vi "4_Wire_Resistance.vi"(6 "Waveform_Template":waveform(dbl), 8 "error in":errorcluster, 11 "DAQ970 in":refnum<class "DAQ970.lvclass">) -> (0 "error out":errorcluster, 2 "Resistive_Measurement":waveform(dbl)[](array[waveform]), 3 "DAQ970 out":refnum<class "DAQ970.lvclass">)   [LabVIEW 2019, in "DAQ970.lvlib" / "DAQ970.lvclass"]
uses:
  Library/DAQ970.lvclass
  Library/DAQ970.lvclass/DAQ970.ctl
  <instrlib>/Keysight DAQ970/Keysight DAQ970.lvlib
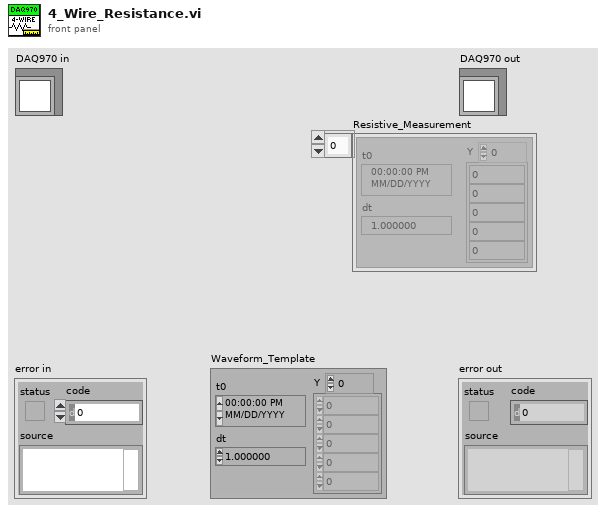
[diagram p1: front panel]
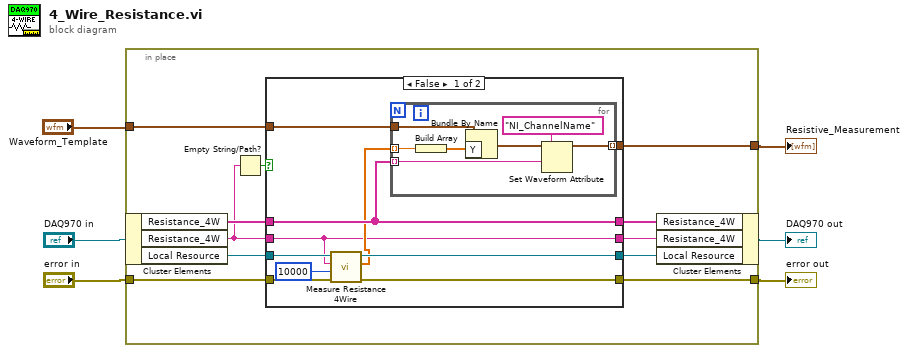
[diagram p0: block diagram]
diagram:
  n1 = in-place {
    in-place-border: "error in" -> [w11]
    in-place-border: [w12] -> w4
    in-place-border: "Waveform_Template" -> [w17]
    in-place-border: [w15] -> w6
    n2 = in-place-cluster #1("DAQ970 in") -> ("Resistance_4W"=w16:string[], "Resistance_4W"=w10:string, "Local Resource"=w14:refnum<k15>)
    n3 = Empty String/Path?(string/path=w10) -> (empty?=w9:bool)
    n4 = case shown="False" w9 {
      tunnel: w17 -> [w27 _]
      tunnel: w16 -> [w25 w38]
      tunnel: [w26 _] -> w15
      tunnel: w14 -> [w24 w36]
      tunnel: [w23 w36] -> w13
      tunnel: [w21 w35] -> w12
      tunnel: w11 -> [w20 w35]
      tunnel: w10 -> [w18 w37]
      tunnel: [w25 w38] -> w8
      tunnel: [w18 w37] -> w7
      frame False {
        n5 = call <instrlib>:"Measure Resistance 4Wire.vi"("error in (no error)"=w20, "MaxTimeMilliseconds"=10000, "ChannelList"=w18, "instrument handle"=w24) -> ("error out"=w21:errorcluster, "Val"=w22:dbl[], "instrument handle out"=w23:refnum<k15>)  [unwired: 4 in, 1 out]
        n6 = for {
          tunnel: w22 -> [w33] mode=indexing
          tunnel: w27 -> [w34]
          tunnel: w25 -> [w29] mode=indexing
          tunnel: [w28] -> w26 mode=indexing
          n7 = Build Array(w33) -> (w32:dbl[])
          n8 = Bundle By Name(cluster=w34, "Y"=w32) -> (w31:waveform(dbl))
          n9 = Set Waveform Attribute(5:w29, 6:"NI_ChannelName" ("name"), 7:w31) -> (3:w28:waveform(dbl))  [unwired: 1 in, 2 out]
        }
      }
      frame True {
      }
    }
    n10 = in-place-cluster #1("Resistance_4W"=w8, "Resistance_4W"=w7, "Local Resource"=w13) -> (→"DAQ970 out":refnum<class "DAQ970.lvclass">)
  }
  "error out" <- w4
  "Resistive_Measurement" <- w6
